vi "Slice Index Array in Contiguous Chunks.vi"(2 "Array in":i32[](array[numeric])) -> (7 "Contiguous sub-Arrays":cluster{"Array":i32[]}[](array[cluster]))   [LabVIEW 2019]
doc: "Sorts the input index array in increasing order and slices it into chunks of consecutive indices."
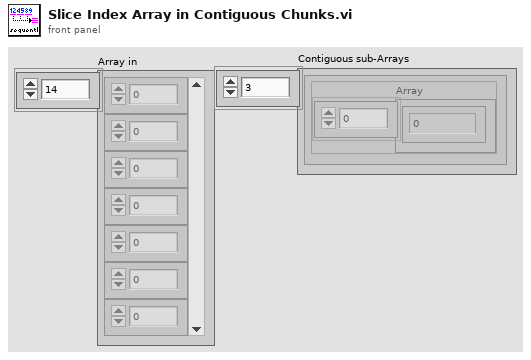
[diagram p1: front panel]
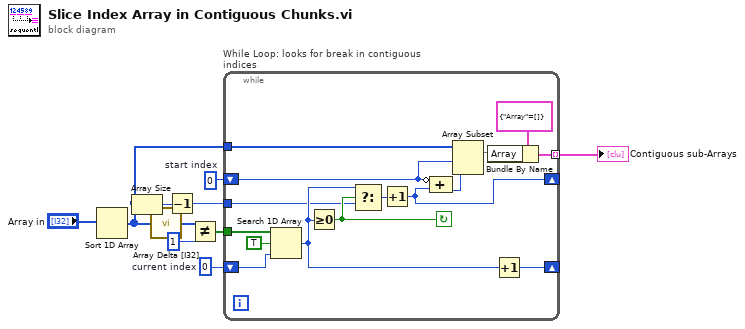
[diagram p0: block diagram]
diagram:
  w4 = 0  # start index
  w6 = 0  # current index
  n1 = Sort 1D Array(array="Array in") -> (sorted array=w3:i32[])
  n2 = Array Size(array=w3) -> (size(s)=w2:i32)
  n3 = call "Array Delta [I32].vi"("Array in"=w3) -> ("Array Delta out"=w9:i32[])  [unwired: 8 in]
  n4 = Decrement(x=w2) -> (x-1=w1:i32)
  n5 = Not Equal?(x=w9, y=1) -> (x != y?=w7:bool[])
  n6 = while "While Loop: looks for break in contiguous indices" {
    tunnel: w7 -> [w25]
    shift-right: [w17] -> _
    shift-left: w6 -> [w23]
    tunnel: w3 -> [w22]
    shift-right: [w11] -> _
    shift-left: w4 -> [w18]
    tunnel: [w19] -> w5 mode=indexing
    tunnel: w1 -> [w13]
    stop <- w15 continue-if-true
    n7 = Search 1D Array(1D array=w25, element=TRUE, start index (0)=w23) -> (index of element=w14:i32)
    n8 = Greater Or Equal To 0?(x=w14) -> (x >= 0?=w15:bool)
    n9 = Select(t=w14, s=w15, f=w13) -> (s? t:f=w12:i32)
    n10 = Increment(x=w12) -> (x+1=w11:i32)
    n11 = Compound Arithmetic op=ADD(invert w18, w11) -> (w16:i32)
    n12 = Array Subset(array=w22, index=w18, length=w16) -> (w20:i32[])
    n13 = Bundle By Name(cluster=cluster{"Array":i32[]} {"Array"=[]} ("Contiguous sub-Arrays"), "Array"=w20) -> (w19:cluster{"Array":i32[]})
    n14 = Increment(x=w14) -> (x+1=w17:i32)
  }
  "Contiguous sub-Arrays" <- w5
